vi "StopSaving.vi"(8 "error in (no error)":errorcluster, 11 "Saving Thread Data in":T1) -> (0 "error out":errorcluster, 3 "Saving Thread Data out":T1)   [LabVIEW 2019]
uses:
  Typedefs/Saving Thread/#cluster_SavingThreadData.ctl
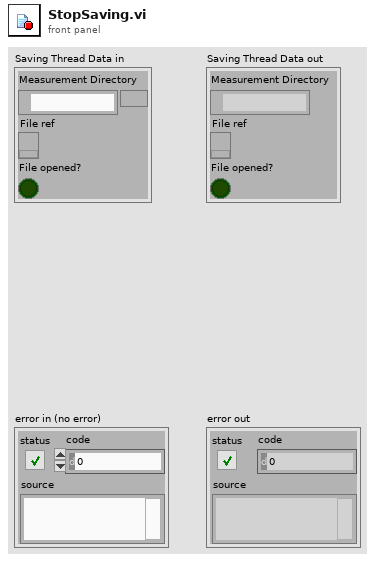
[diagram p1: front panel]
types:
  T1 = typedef "#cluster_SavingThreadData.ctl" = cluster{"Measurement Directory":path, "File ref":refnum<k34>, "File opened?":bool}
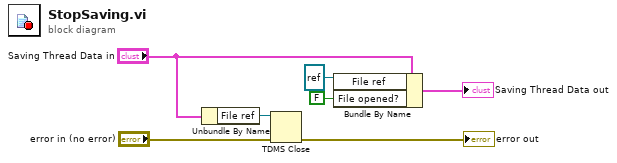
[diagram p0: block diagram]
diagram:
  n1 = Unbundle By Name("Saving Thread Data in") -> ("File ref"=w4:refnum<k34>)
  n2 = TDMS Close(8:"error in (no error)", 11:w4) -> (0:→"error out":errorcluster)  [unwired: 1 out]
  n3 = Bundle By Name(cluster="Saving Thread Data in", "File ref"=refnum<k34> refnum, "File opened?"=FALSE) -> (→"Saving Thread Data out":T1)
